vi "ServoControl.vi"(10 "Servo data in":T1) -> ()   [LabVIEW 2023]
uses:
  controls/ServoData.ctl
panel:
  out "Servo data out":T1
  in  "Stop Button":bool
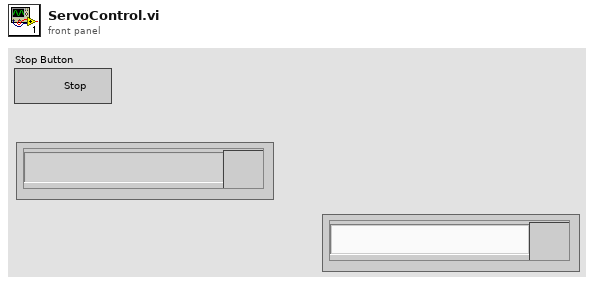
[diagram p1: front panel]
types:
  T1 = typedef "ServoData.ctl" = cluster{"Name":string, "Channel":u8, "Delete Button":bool}
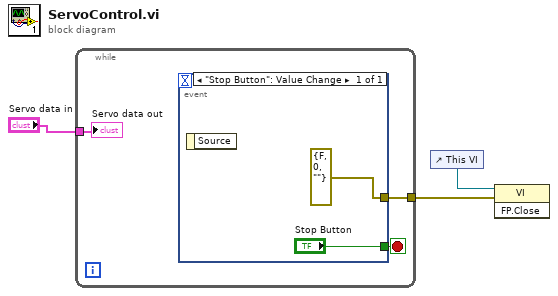
[diagram p0: block diagram]
diagram:
  n1 = while {
    tunnel: "Servo data in" -> [w4]
    tunnel: [w5] -> w1
    stop <- w6 stop-if-true
    n2 = event shown="[0] \"Stop Button\": Value Change" {
      selector: _ -> [_]
      dyn-events: _ -> [_]
      timeout: _ -> [_]
      tunnel: ["Stop Button"] -> w6
      tunnel: [errorcluster {"status"=FALSE, "code"=0, "source"=""} ("error in (no error)")] -> w5
      event "Stop Button": Value Change {
        n3 = event-data() -> ()  [unwired: 1 in, 1 out]
      }
    }
    "Servo data out" <- w4
  }
  n4 = control-ref of="This VI"() -> (w2:refnum<vi>)
  n5 = invoke class="VI" method="FP.Close"(reference=w2, error in=w1) -> ()  [unwired: 1 in, 3 out]
